vi "mod_stuApa.vi"(5 "connection reference":T3) -> ()   [LabVIEW 2018]
uses:
  <vilib>/addons/database/Connection.llb/Conn ObjectReference.ctl
  <vilib>/addons/database/Connection.llb/Conn Execute.vi
  <vilib>/addons/database/Recordset.llb/Rec Fetch Recordset Data (R).vi
  <vilib>/addons/database/_DB Variant To Data/Database Variant To Data.xnode
  <vilib>/addons/database/NI_Database_API.lvlib
panel:
  in  "表名":string="sa_room_electricity_Info"
  in  "表字段类型簇":T1
  out "数组":string[](array[string])
  in  "字段名数组":string[](array[string])=["apartmentNamegyc", "roomIDgyc", "usedFeegyc", "remainingFeegyc"]
  out "error out":errorcluster
  in  "修改按钮":bool
  in  "清除指示灯":bool
  in  "添加按钮":bool
  in  "删除按钮":bool
  in  "查询按钮":bool
  in  "信息输入框":T2
  in  "刷新按钮":bool
  in  "信息框":i32(listbox)
  in  "已编辑行数组":u32[](array[numeric])
  in  "信息框缓冲备份":string[][](array[string])
  in  "error in (no error)":errorcluster
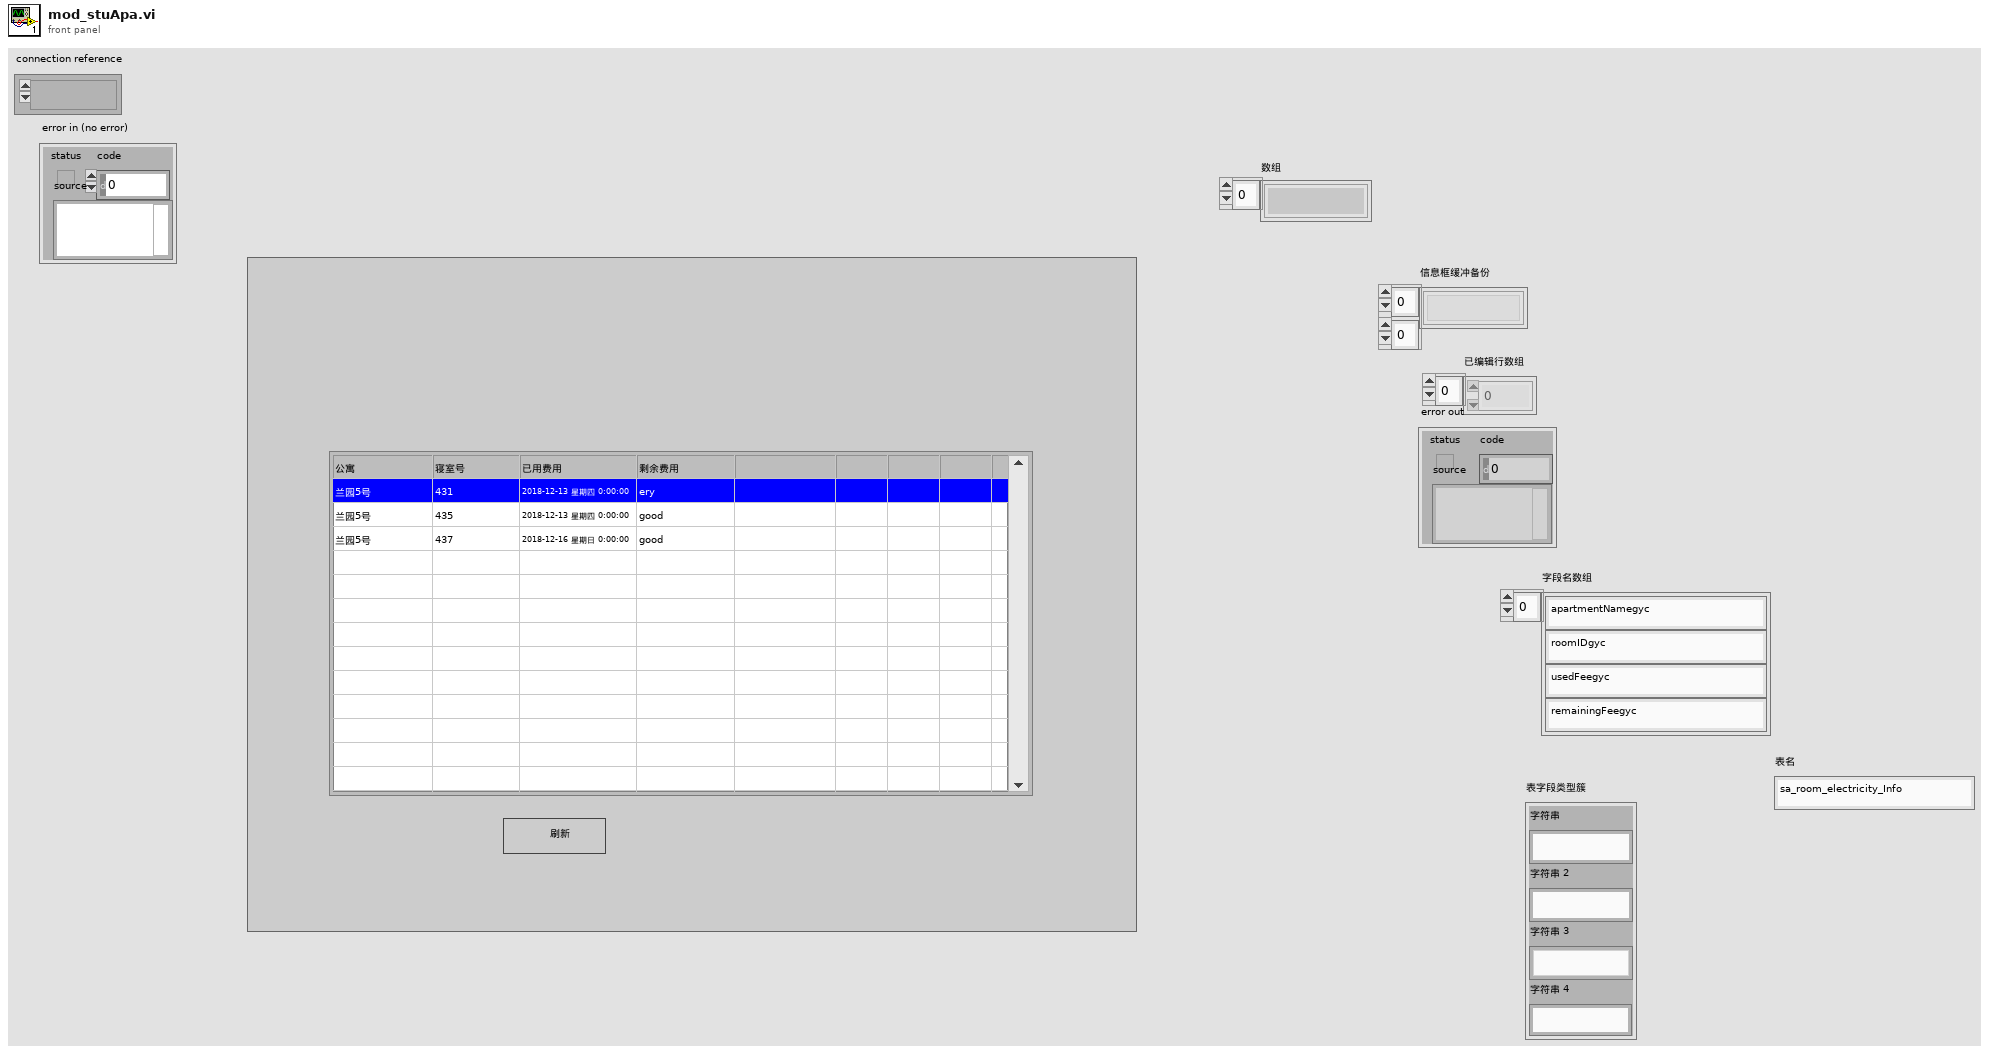
[diagram p1: front panel]
types:
  T1 = cluster{"字符串":string, "字符串 2":string, "字符串 3":string, "字符串 4":string}
  T2 = cluster{"公寓":string, "寝室号":string, "已用费用":string, "剩余费用":string}
  T3 = typedef "NI_Database_API.lvlib/Conn ObjectReference.ctl" = refnum<k1>
  T4 = typedef "NI_Database_API.lvlib/Rec ObjectReference.ctl" = refnum<k1>
  T5 = cluster{string, string, string, string, string}[]
  T6 = typedef "LVPoint32TypeDef.ctl" = cluster{"Horizontal":i32, "Vertical":i32}
  T7 = typedef "LVRowAndColumnTypeDef.ctl" = cluster{"Row":i32, "Column":i32}
  T8 = cluster{"字符串":string, "字符串 2":string, "字符串 3":string, "字符串 4":string}[]
  T9 = cluster{"[0]":string, "[1]":string, "[2]":string, "[3]":string}
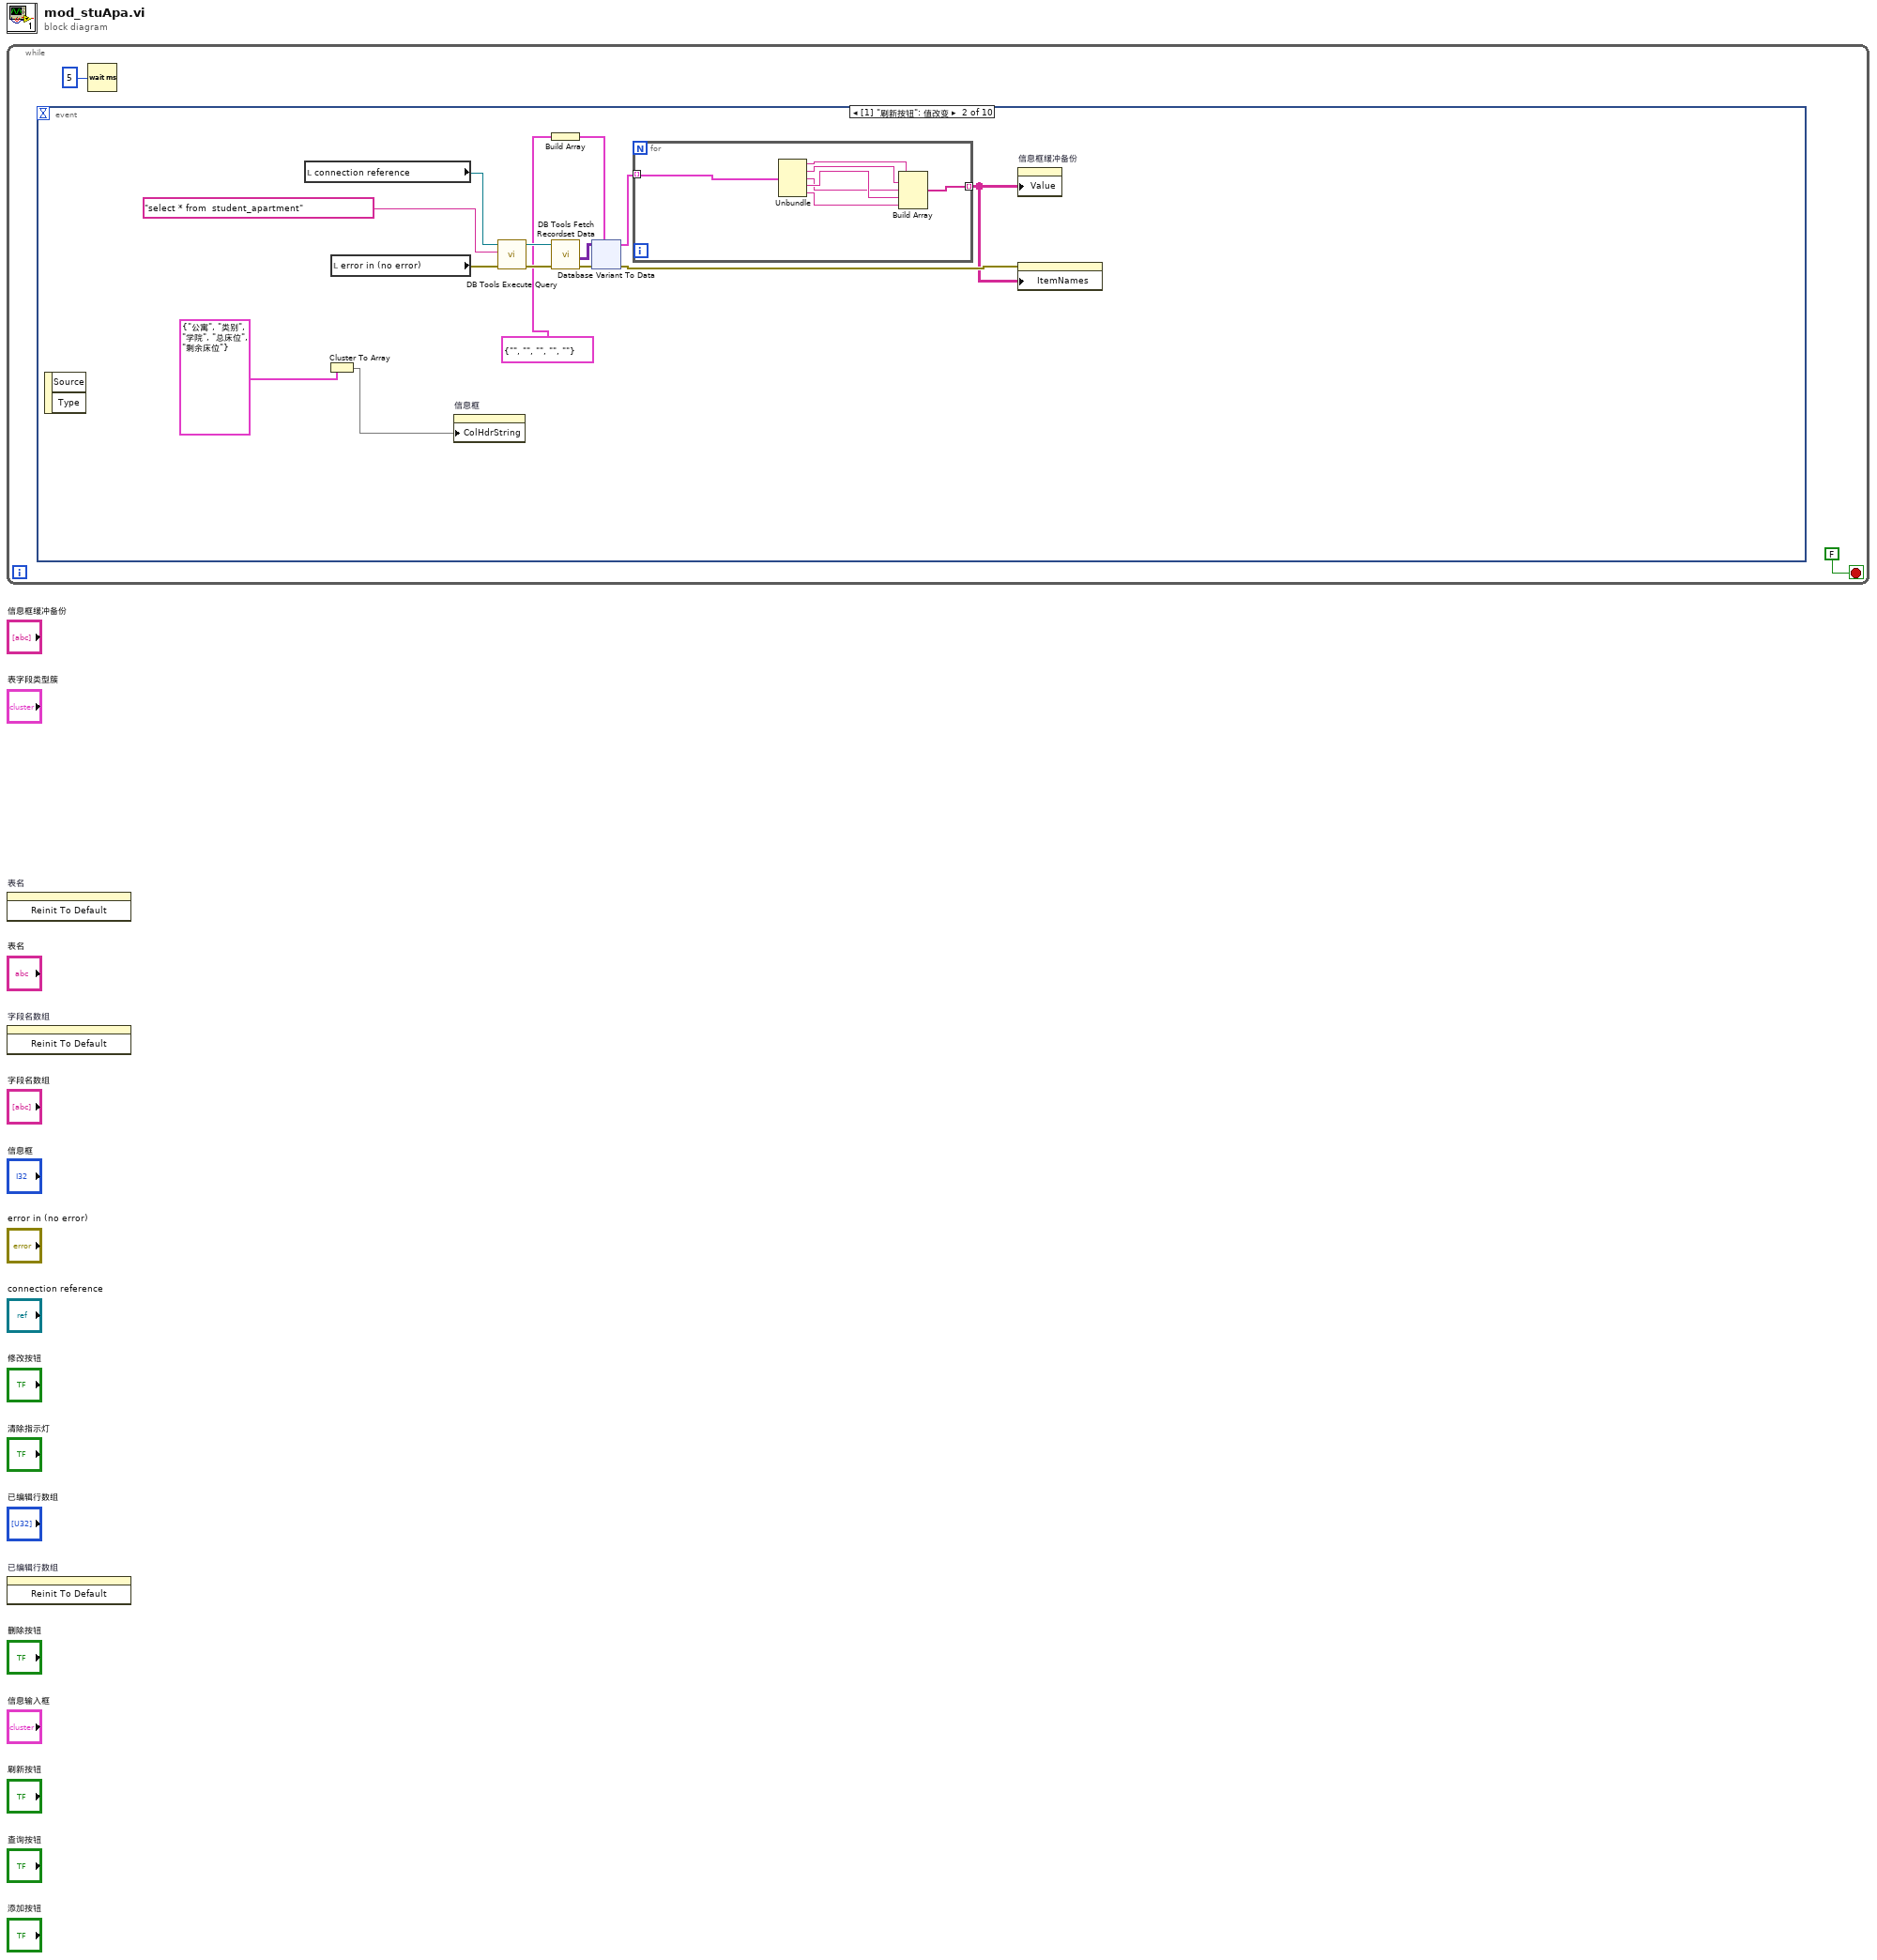
[diagram p0: block diagram]
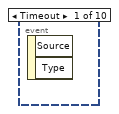
[diagram p2: hidden frame]
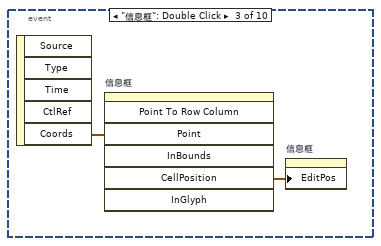
[diagram p3: hidden frame]
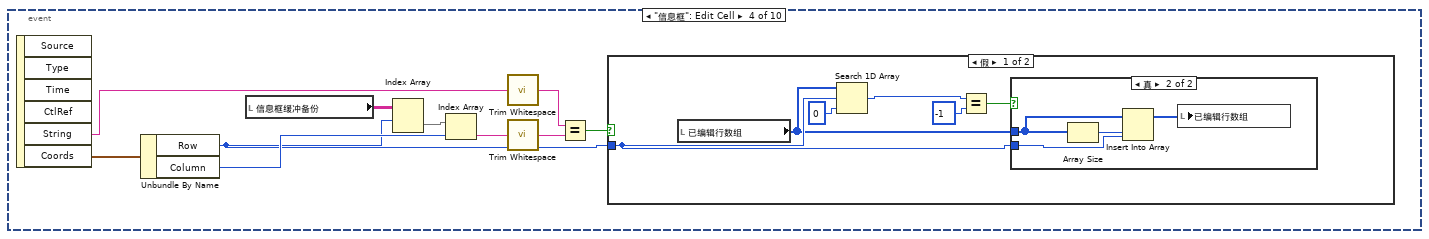
[diagram p4: hidden frame]
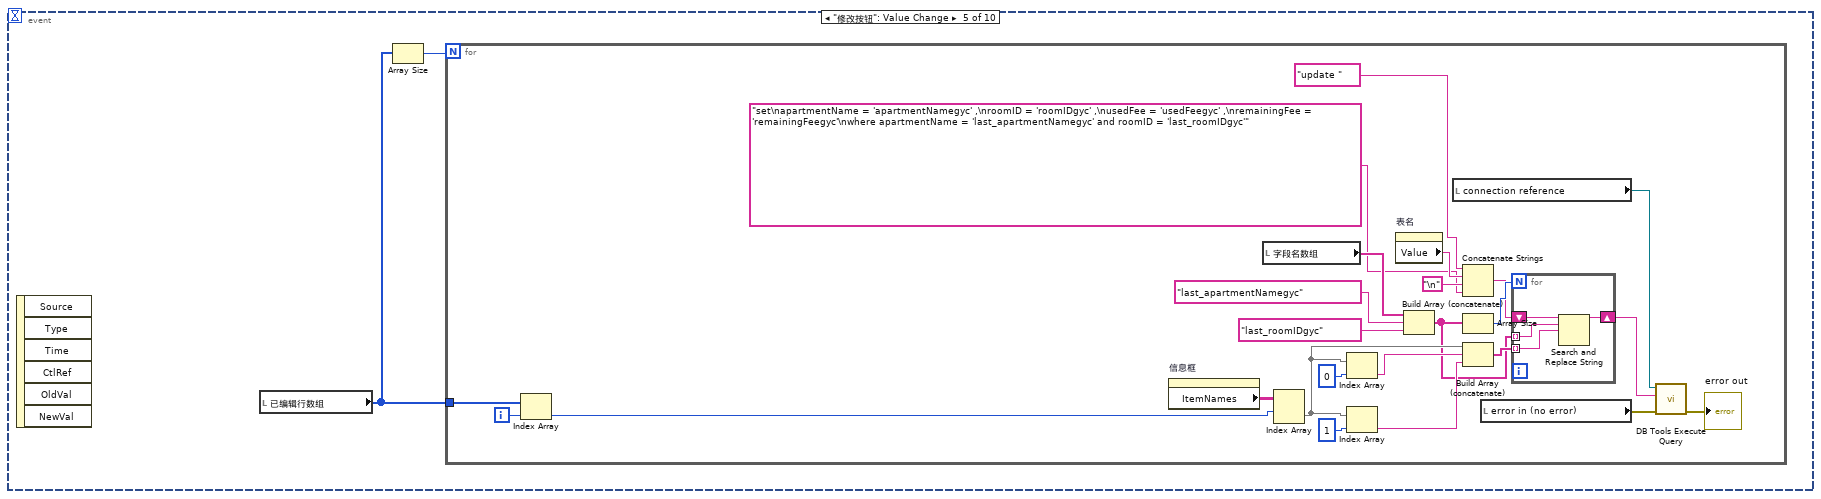
[diagram p7: hidden frame]
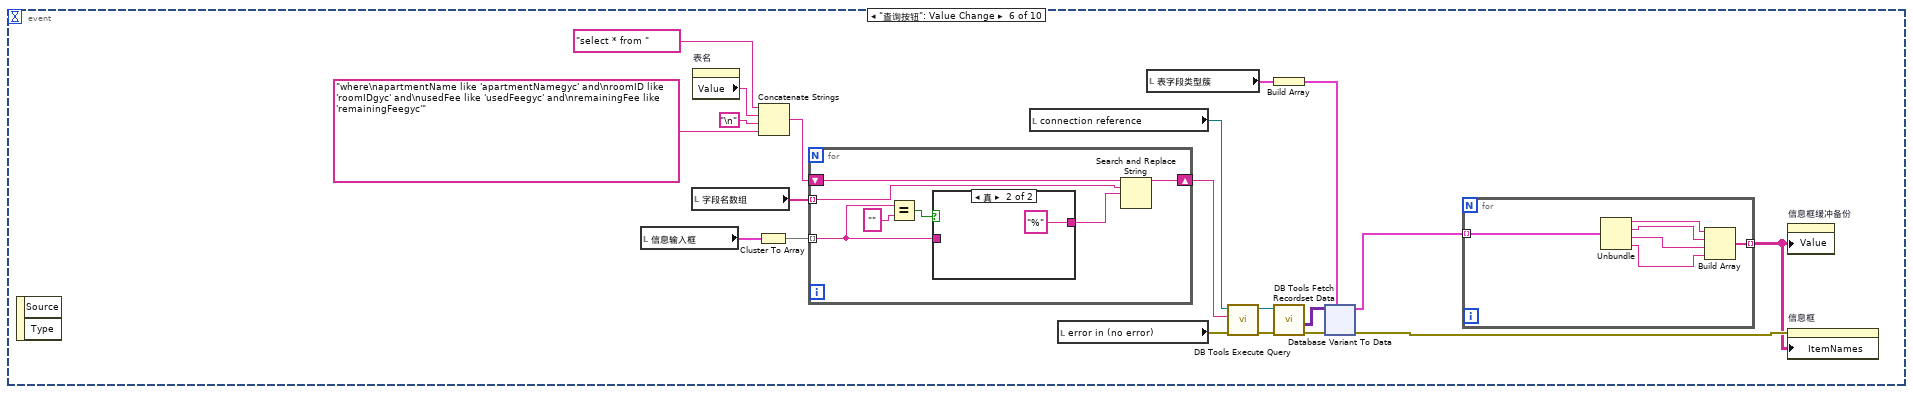
[diagram p8: hidden frame]
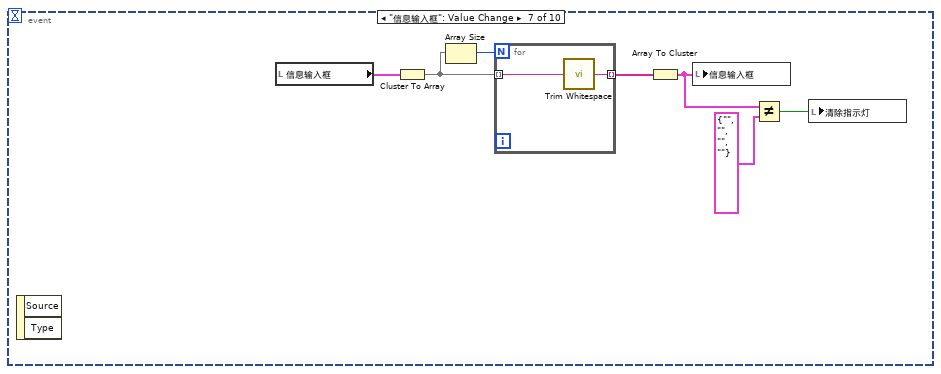
[diagram p10: hidden frame]
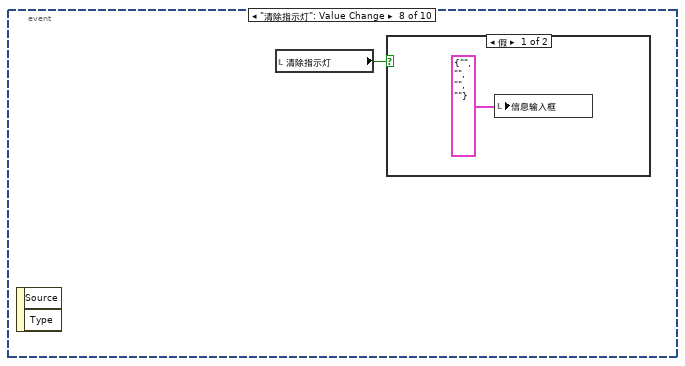
[diagram p11: hidden frame]
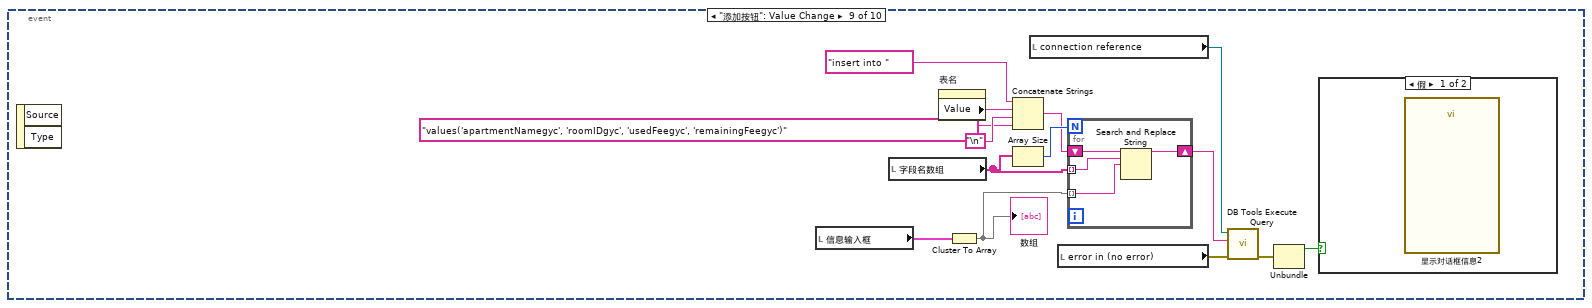
[diagram p13: hidden frame]
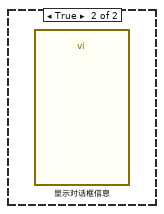
[diagram p14: hidden frame]
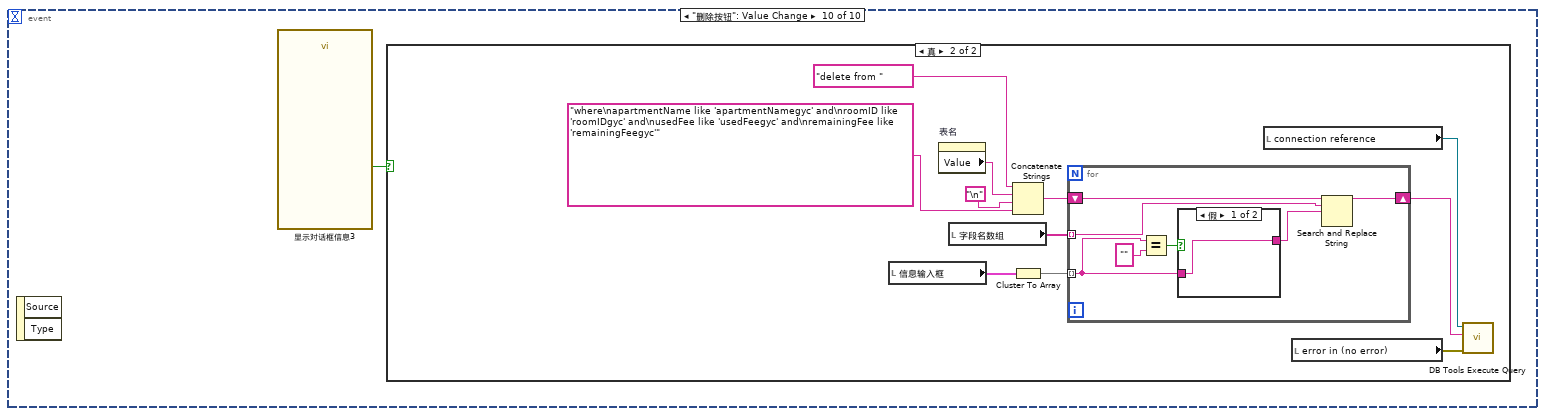
[diagram p15: hidden frame]
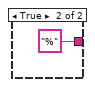
[diagram p17: hidden frame]
diagram:
  n1 = while {
    stop <- FALSE stop-if-true
    n2 = event shown="[1] \"刷新按钮\": 值改变" {
      selector: _ -> [_ _ _ _ _ _ _ _ _ _]
      dyn-events: _ -> [_ _ _ _ _ _ _ _ _ _]
      timeout: _ -> [_ _ _ _ _ _ _ _ _ _]
      event Timeout {
        n3 = event-data() -> ()  [unwired: 1 in, 2 out]
      }
      event "刷新按钮": Value Change {
        n4 = event-data() -> ()  [unwired: 1 in, 2 out]
        n5 = local read "connection reference"() -> (w9:T3)
        n6 = Cluster To Array(cluster=cluster{string, string, string, string, string} {"公寓", "类别", "学院", "总床位", "剩余床位"}) -> (array=w4:string[])
        n7 = local read "error in (no error)"() -> (w8:errorcluster)
        n8 = property on="信息框" class="MCListbox (严格)"("ColHdrString"=w4) -> ()  [unwired: 2 in, 2 out]
        n9 = call-poly <vilib>:"DB Tools Execute Query.vi"("error in (no error)"=w8, "SQL query"="select * from  student_apartment", "connection reference"=w9) -> ("error out"=w11:errorcluster, "recordset reference"=w10:T4)  [unwired: 5 in]
        n10 = Build Array(cluster{string, string, string, string, string} {"", "", "", "", ""}) -> (w14:T5)
        n11 = call-poly <vilib>:"DB Tools Fetch Recordset Data.vi"("error in (no error)"=w11, "recordset reference"=w10) -> ("error out"=w12:errorcluster, "recordset data"=w13:variant[][])  [unwired: 3 in, 1 out]
        n12 = xnode "Database Variant To Data"("database variant"=w13, "error in (no error)"=w12, "type"=w14) -> ("data"=w15:T5, "error out"=w16:errorcluster)
        n13 = for {
          tunnel: w15 -> [w23] mode=indexing
          tunnel: [w19] -> w7 mode=indexing
          n14 = Unbundle(w23) -> (w22:string, w21:string, w18:string, w20:string, w17:string)
          n15 = Build Array(w22, w21, w18, w20, w17) -> (w19:string[])
        }
        n16 = property on="信息框缓冲备份" class="Arr (严格)"("Value"=w7) -> ()  [unwired: 2 in, 2 out]
        n17 = property on="信息框" class="MCListbox (严格)"(error in=w16, "ItemNames"=w7) -> ()  [unwired: 1 in, 2 out]
      }
      event "信息框": Double Click {
        n18 = event-data() -> ("Coords"=w190:T6)  [unwired: 1 in, 4 out]
        n19 = invoke on="信息框" class="MCListbox (严格)" method="Point To Row Column"("Point"=w190) -> ("CellPosition"=w189:T7)  [unwired: 6 in, 6 out]
        n20 = property on="信息框" class="MCListbox (严格)"("EditPos"=w189) -> ()  [unwired: 2 in, 2 out]
      }
      event "信息框": Edit Cell {
        n21 = event-data() -> ("String"=w195:string, "Coords"=w196:T7)  [unwired: 1 in, 4 out]
        n22 = Unbundle By Name(w196) -> ("Row"=w198:i32, "Column"=w200:i32)
        n23 = local read "信息框缓冲备份"() -> (w197:string[][])
        n24 = Index Array(array=w197, index (row)=w198) -> (element=w199:string[])  [unwired: 1 in]
        n25 = Index Array(array=w199, index=w200) -> (element=w193:string)
        n26 = call <vilib>:"Trim Whitespace.vi"("string"=w195) -> ("trimmed string"=w194:string)  [unwired: 1 in]
        n27 = call <vilib>:"Trim Whitespace.vi"("string"=w193) -> ("trimmed string"=w192:string)  [unwired: 1 in]
        n28 = Equal?(x=w194, y=w192) -> (x = y?=w191:bool)
        n29 = case shown="假" w191 {
          tunnel: w198 -> [w206 _]
          frame False {
            n30 = local read "已编辑行数组"() -> (w204:u32[])
            n31 = Search 1D Array(1D array=w204, element=w206, start index (0)=0 ("开始索引(0)")) -> (index of element=w205:i32)
            n32 = Equal?(x=w205, y=-1) -> (x = y?=w203:bool)
            n33 = case shown="真" w203 {
              tunnel: w204 -> [_ w208]
              tunnel: w206 -> [_ w210]
              frame False {
              }
              frame True {
                n34 = Array Size(array=w208) -> (size(s)=w207:i32)
                n35 = Insert Into Array(array=w208, index=w207, new element=w210) -> (w209:u32[])
                n36 = local write "已编辑行数组"(w209) -> ()
              }
            }
          }
          frame True {
          }
        }
      }
      event "修改按钮": Value Change {
        n37 = event-data() -> ()  [unwired: 1 in, 6 out]
        n38 = local read "已编辑行数组"() -> (w212:u32[])
        n39 = Array Size(array=w212) -> (size(s)=w211:i32)
        n40 = for {
          N: w211 -> [_]
          tunnel: w212 -> [w233]
          i -> [w234]
          n41 = Index Array(array=w233, index=w234) -> (element=w235:u32)
          n42 = property on="信息框" class="MCListbox (严格)"() -> ("ItemNames"=w236:string[][])  [unwired: 2 in, 2 out]
          n43 = local read "字段名数组"() -> (w218:string[])
          n44 = Index Array(array=w236, index (row)=w235) -> (element=w226:string[])  [unwired: 1 in]
          n45 = Index Array(array=w226, index=0 ("索引")) -> (element=w228:string)
          n46 = Index Array(array=w226, index=1 ("索引")) -> (element=w225:string)
          n47 = property on="表名" class="Str"() -> ("Value"=w215:string)  [unwired: 2 in, 2 out]
          n48 = Build Array (concatenate)(w218, "last_apartmentNamegyc" ("字符串"), "last_roomIDgyc" ("字符串")) -> (w221:string[])
          n49 = local read "connection reference"() -> (w232:T3)
          n50 = Concatenate Strings("update ", w215, "\n", "set\napartmentName = 'apartmentNamegyc' ,\nroomID = 'roomIDgyc' ,\nusedFee = 'usedFeegyc' ,\nremainingFee = 'remainingFeegyc'\nwhere apartmentName = 'last_apartmentNamegyc' and roomID = 'last_roomIDgyc'") -> (w217:string)
          n51 = Array Size(array=w221) -> (size(s)=w220:i32)
          n52 = Build Array (concatenate)(w226, w228, w225) -> (w222:string[])
          n53 = local read "error in (no error)"() -> (w231:errorcluster)
          n54 = for {
            N: w220 -> [_]
            shift-right: [w239] -> w219
            shift-left: w217 -> [w240]
            tunnel: w222 -> [w238] mode=indexing
            tunnel: w221 -> [w237] mode=indexing
            n55 = Search and Replace String(input string=w240, search string=w237, replace string=w238) -> (result string=w239:string)  [unwired: 5 in, 3 out]
          }
          n56 = call-poly <vilib>:"DB Tools Execute Query.vi"("error in (no error)"=w231, "SQL query"=w219, "connection reference"=w232) -> ("error out"=→"error out":errorcluster)  [unwired: 5 in, 1 out]
        }
      }
      event "查询按钮": Value Change {
        n57 = event-data() -> ()  [unwired: 1 in, 2 out]
        n58 = local read "信息输入框"() -> (w249:T2)
        n59 = local read "字段名数组"() -> (w247:string[])
        n60 = property on="表名" class="Str"() -> ("Value"=w244:string)  [unwired: 2 in, 2 out]
        n61 = Cluster To Array(cluster=w249) -> (array=w248:string[])
        n62 = Concatenate Strings("select * from ", w244, "\n", "where\napartmentName like 'apartmentNamegyc' and\nroomID like 'roomIDgyc' and\nusedFee like 'usedFeegyc' and\nremainingFee like 'remainingFeegyc'") -> (w245:string)
        n63 = for {
          shift-right: [w266] -> w250
          shift-left: w245 -> [w267]
          tunnel: w247 -> [w263] mode=indexing
          tunnel: w248 -> [w262] mode=indexing
          n64 = Equal?(x=w262, y="") -> (x = y?=w265:bool)
          n65 = case shown="真" w265 {
            tunnel: [w268 "%"] -> w261
            tunnel: w262 -> [w268 _]
            frame False {
            }
            frame True {
            }
          }
          n66 = Search and Replace String(input string=w267, search string=w263, replace string=w261) -> (result string=w266:string)  [unwired: 5 in, 3 out]
        }
        n67 = local read "connection reference"() -> (w260:T3)
        n68 = local read "error in (no error)"() -> (w259:errorcluster)
        n69 = local read "表字段类型簇"() -> (w246:T1)
        n70 = call-poly <vilib>:"DB Tools Execute Query.vi"("error in (no error)"=w259, "SQL query"=w250, "connection reference"=w260) -> ("error out"=w252:errorcluster, "recordset reference"=w253:T4)  [unwired: 5 in]
        n71 = Build Array(w246) -> (w256:T8)
        n72 = call-poly <vilib>:"DB Tools Fetch Recordset Data.vi"("error in (no error)"=w252, "recordset reference"=w253) -> ("error out"=w254:errorcluster, "recordset data"=w255:variant[][])  [unwired: 3 in, 1 out]
        n73 = xnode "Database Variant To Data"("database variant"=w255, "error in (no error)"=w254, "type"=w256) -> ("data"=w257:T8, "error out"=w258:errorcluster)
        n74 = for {
          tunnel: w257 -> [w274] mode=indexing
          tunnel: [w275] -> w251 mode=indexing
          n75 = Unbundle(w274) -> ("字符串"=w273:string, "字符串 2"=w272:string, "字符串 3"=w270:string, "字符串 4"=w271:string)
          n76 = Build Array(w273, w272, w270, w271) -> (w275:string[])
        }
        n77 = property on="信息框缓冲备份" class="Arr (严格)"("Value"=w251) -> ()  [unwired: 2 in, 2 out]
        n78 = property on="信息框" class="MCListbox (严格)"(error in=w258, "ItemNames"=w251) -> ()  [unwired: 1 in, 2 out]
      }
      event "信息输入框": Value Change {
        n79 = event-data() -> ()  [unwired: 1 in, 2 out]
        n80 = local read "信息输入框"() -> (w413:T2)
        n81 = Cluster To Array(cluster=w413) -> (array=w412:string[])
        n82 = Array Size(array=w412) -> (size(s)=w414:i32)
        n83 = for {
          N: w414 -> [_]
          tunnel: w412 -> [w418] mode=indexing
          tunnel: [w417] -> w411 mode=indexing
          n84 = call <vilib>:"Trim Whitespace.vi"("string"=w418) -> ("trimmed string"=w417:string)  [unwired: 1 in]
        }
        n85 = Array To Cluster(array=w411) -> (cluster=w410:T9)
        n86 = local write "信息输入框"(w410) -> ()
        n87 = Not Equal?(x=w410, y=cluster{string, string, string, string} {"", "", "", ""}) -> (x != y?=w415:bool)
        n88 = local write "清除指示灯"(w415) -> ()
      }
      event "清除指示灯": Value Change {
        n89 = event-data() -> ()  [unwired: 1 in, 2 out]
        n90 = local read "清除指示灯"() -> (w419:bool)
        n91 = case shown="假" w419 {
          frame False {
            n92 = local write "信息输入框"(cluster{string, string, string, string} {"", "", "", ""}) -> ()
          }
          frame True {
          }
        }
      }
      event "添加按钮": Value Change {
        n93 = event-data() -> ()  [unwired: 1 in, 2 out]
        n94 = local read "信息输入框"() -> (w429:T2)
        n95 = local read "字段名数组"() -> (w427:string[])
        n96 = property on="表名" class="Str"() -> ("Value"=w423:string)  [unwired: 2 in, 2 out]
        n97 = Cluster To Array(cluster=w429) -> (array=w428:string[])
        "数组" <- w428
        n98 = Concatenate Strings("insert into " ("SQL query"), w423, "\n", "values('apartmentNamegyc', 'roomIDgyc', 'usedFeegyc', 'remainingFeegyc')") -> (w425:string)
        n99 = Array Size(array=w427) -> (size(s)=w430:i32)
        n100 = local read "connection reference"() -> (w433:T3)
        n101 = local read "error in (no error)"() -> (w434:errorcluster)
        n102 = for {
          N: w430 -> [_]
          shift-right: [w438] -> w426
          shift-left: w425 -> [w437]
          tunnel: w428 -> [w436] mode=indexing
          tunnel: w427 -> [w435] mode=indexing
          n103 = Search and Replace String(input string=w437, search string=w435, replace string=w436) -> (result string=w438:string)  [unwired: 5 in, 3 out]
        }
        n104 = call-poly <vilib>:"DB Tools Execute Query.vi"("error in (no error)"=w434, "SQL query"=w426, "connection reference"=w433) -> ("error out"=w432:errorcluster)  [unwired: 5 in, 1 out]
        n105 = Unbundle(w432) -> ("status"=w431:bool)  [unwired: 2 out]
        n106 = case shown="假" w431 {
          frame False {
            n107 = call "显示对话框信息2"() -> ()  [unwired: 10 in, 2 out]
          }
          frame True {
            n108 = call "显示对话框信息"() -> ()  [unwired: 10 in, 2 out]
          }
        }
      }
      event "删除按钮": Value Change {
        n109 = event-data() -> ()  [unwired: 1 in, 2 out]
        n110 = call "显示对话框信息3"() -> ("确定"=w439:bool)  [unwired: 10 in, 1 out]
        n111 = case shown="真" w439 {
          frame False {
          }
          frame True {
            n112 = local read "信息输入框"() -> (w446:T2)
            n113 = property on="表名" class="Str"() -> ("Value"=w440:string)  [unwired: 2 in, 2 out]
            n114 = local read "字段名数组"() -> (w445:string[])
            n115 = Concatenate Strings("delete from ", w440, "\n", "where\napartmentName like 'apartmentNamegyc' and\nroomID like 'roomIDgyc' and\nusedFee like 'usedFeegyc' and\nremainingFee like 'remainingFeegyc'") -> (w444:string)
            n116 = Cluster To Array(cluster=w446) -> (array=w447:string[])
            n117 = for {
              tunnel: w447 -> [w454] mode=indexing
              tunnel: w445 -> [w453] mode=indexing
              shift-right: [w451] -> w448
              shift-left: w444 -> [w452]
              n118 = Equal?(x=w454, y="") -> (x = y?=w456:bool)
              n119 = case shown="假" w456 {
                tunnel: [w458 "%"] -> w455
                tunnel: w454 -> [w458 _]
                frame False {
                }
                frame True {
                }
              }
              n120 = Search and Replace String(input string=w452, search string=w453, replace string=w455) -> (result string=w451:string)  [unwired: 5 in, 3 out]
            }
            n121 = local read "connection reference"() -> (w449:T3)
            n122 = local read "error in (no error)"() -> (w450:errorcluster)
            n123 = call-poly <vilib>:"DB Tools Execute Query.vi"("error in (no error)"=w450, "SQL query"=w448, "connection reference"=w449) -> ()  [unwired: 5 in, 2 out]
          }
        }
      }
    }
    n124 = Wait (ms)(milliseconds to wait=u32 5 ("等待时间（毫秒）")) -> ()  [unwired: 1 out]
  }
  n125 = invoke on="表名" class="Str" method="Reinit To Default"() -> ()  [unwired: 3 in, 3 out]
  n126 = invoke on="字段名数组" class="Arr (严格)" method="Reinit To Default"() -> ()  [unwired: 3 in, 3 out]
  n127 = invoke on="已编辑行数组" class="Arr (严格)" method="Reinit To Default"() -> ()  [unwired: 3 in, 3 out]
